vi "Configure Multi Eval Meas List Segment Sequence Generation.vi"(0 "VISA resource name":refnum<visa-resource-name>, 1 "Allocation (1)":T1=1, 2 "DMRS ID (0)":i32, 5 "Instance (1)":T4=1, 7 "Segment (1)":T3=1, 9 "Carrier Component (1)":T2=1, 11 "error in (no error)":errorcluster, 12 "Initialization (Cell ID Used)":i32(ring) items=["Cell ID Used", "DMRS ID Used"], 13 "nSCID (0)":i32) -> (4 "VISA resource name out":refnum<visa-resource-name>, 15 "error out":errorcluster)   [LabVIEW 2020, in "Rohde&Schwarz CMXP NR FR2 Measurement.lvlib"]
doc: "Configures the initialization of the DM-RS sequence generation, for carrier <cc>, allocation <a> in segment <no>.\n\nAttribute:\nRSCMXPNRFR2M_ATTR_MULTI_EVAL_MEASUREMENT_LIST_SEGMENT_SEQUENCE_GENERATION\n\nRemote-control command:\nCONFigure:NRMMw:MEAS<i>:LIST:SEGMent<no>[:CC<cc>]:ALLocation<a>:PUSCh:SGENeration"
uses:
  <instrlib>/Rohde&Schwarz CMXP NR FR2 Measurement/Rohde&Schwarz CMXP NR FR2 Measurement.lvlib
  <instrlib>/Rohde&Schwarz CMXP NR FR2 Measurement/Private/_Instance.ctl
  <instrlib>/Rohde&Schwarz CMXP NR FR2 Measurement/Private/_Segment.ctl
  <instrlib>/Rohde&Schwarz CMXP NR FR2 Measurement/Private/_Carrier Component.ctl
  <instrlib>/Rohde&Schwarz CMXP NR FR2 Measurement/Private/_Allocation.ctl
  <instrlib>/Rohde&Schwarz CMXP NR FR2 Measurement/Private/rsidr_core.llb/rsidr_core.lvlib
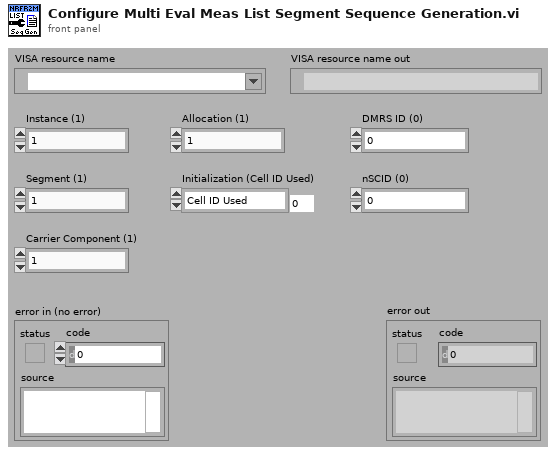
[diagram p1: front panel]
types:
  T1 = typedef "Rohde&Schwarz CMXP NR FR2 Measurement.lvlib/_Allocation.ctl" = i32
  T2 = typedef "Rohde&Schwarz CMXP NR FR2 Measurement.lvlib/_Carrier Component.ctl" = i32
  T3 = typedef "Rohde&Schwarz CMXP NR FR2 Measurement.lvlib/_Segment.ctl" = i32
  T4 = typedef "Rohde&Schwarz CMXP NR FR2 Measurement.lvlib/_Instance.ctl" = i32
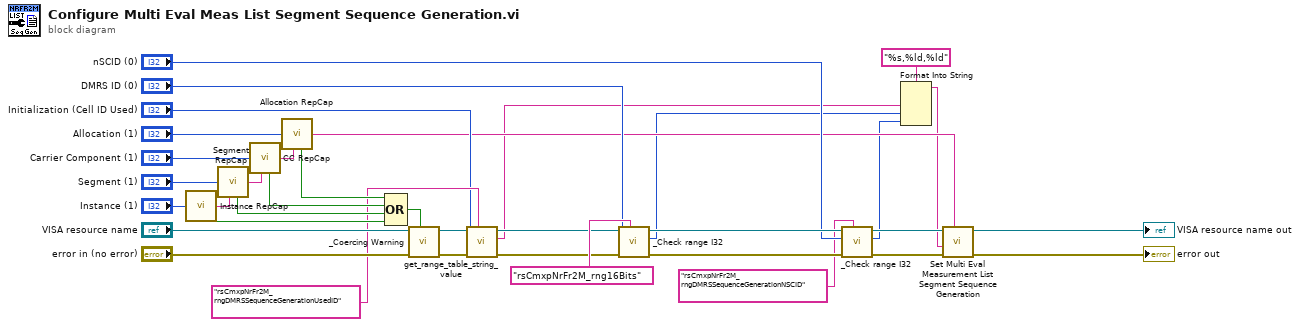
[diagram p0: block diagram]
diagram:
  n1 = call <instrlib>:"Instance RepCap.vi"("Instance In"="Instance (1)") -> ("In Range?"=w30:bool, "RepCap Identifier Out"=w2:string)  [unwired: 1 in]
  n2 = call <instrlib>:"Segment RepCap.vi"("Segment In"="Segment (1)", "RepCap String In (\"\")"=w2) -> ("In Range?"=w29:bool, "RepCap Identifier Out"=w28:string)
  n3 = call <instrlib>:"CC RepCap.vi"("CC In"="Carrier Component (1)", "RepCap String In (\"\")"=w28) -> ("In Range?"=w27:bool, "RepCap Identifier Out"=w26:string)
  n4 = call <instrlib>:"Allocation RepCap.vi"("Allocation In"="Allocation (1)", "RepCap String In (\"\")"=w26) -> ("In Range?"=w25:bool, "RepCap Identifier Out"=w12:string)
  n5 = Compound Arithmetic op=OR(w25, w27, w29, w30) -> (w33:bool)
  n6 = call <instrlib>:"_Coercing Warning.vi"("In Range?"=w33, "error in (no error)"="error in (no error)", "VISA resource name"="VISA resource name") -> ("error out"=w17:errorcluster, "VISA resource name out"=w16:refnum<visa-resource-name>)  [unwired: 7 in]
  n7 = call <instrlib>:"get_range_table_string_value.vi"("Range Table ID in"="rsCmxpNrFr2M_rngDMRSSequenceGenerationUsedID", "error in"=w17, "I32 input"="Initialization (Cell ID Used)", "VISA resource name"=w16) -> ("error out"=w21:errorcluster, "String Value out"=w6:string, "VISA resource name out"=w22:refnum<visa-resource-name>)  [unwired: 5 in]
  n8 = call <instrlib>:"_Check range I32.vi"("Range Table Identifier"="rsCmxpNrFr2M_rng16Bits", "error in (no error)"=w21, "I32 Value In"="DMRS ID (0)", "VISA resource name"=w22) -> ("error out"=w18:errorcluster, "I32 Value Out"=w5:i32, "VISA resource name out"=w19:refnum<visa-resource-name>)  [unwired: 5 in]
  n9 = call <instrlib>:"_Check range I32.vi"("Range Table Identifier"="rsCmxpNrFr2M_rngDMRSSequenceGenerationNSCID", "error in (no error)"=w18, "I32 Value In"="nSCID (0)", "VISA resource name"=w19) -> ("error out"=w11:errorcluster, "I32 Value Out"=w4:i32, "VISA resource name out"=w10:refnum<visa-resource-name>)  [unwired: 5 in]
  n10 = Format Into String(format string="%s,%ld,%ld", w6, w5, w4) -> (resulting string=w1:string)  [unwired: 2 in, 1 out]
  n11 = call "Set Multi Eval Measurement List Segment Sequence Generation"("Repeated Capabilities"=w12, "error in (no error)"=w11, "Multi Eval Measurement List Segment Sequence Generation ()"=w1, "instrument handle"=w10) -> ("error out"=→"error out":errorcluster, "instrument handle out"=→"VISA resource name out":refnum<visa-resource-name>)  [unwired: 6 in]
